vi "Add Crank Cam RTM Dependency.vi"(8 "error in (no error)":errorcluster, 9 "Menu hierarchy in":string[](array[string]), 11 "Node Ptr":u64 format="%.0x") -> (0 "error out":errorcluster, 1 "Menu hierarchy out":string[](array[string]), 3 "Action":T1)   [LabVIEW 2011, in "Engine Sim System Explorer.lvlib"]
uses:
  Engine Sim System Explorer.lvlib
  <vilib>/NI Veristand/Custom Device API/Custom Device RTM Dependency.ctl
  TypeDefs/NTeethComp.ctl
  TypeDefs/FullyCustomComp.ctl
  Shared/FullyCustomCommMode.ctl
  TypeDefs/FullyCustomProfilesComp.ctl
  Shared/Engine Simulation Global.vi
  <vilib>/NI Veristand/Custom Device API/Get Item Property (Variant).vi
  <vilib>/NI Veristand/Custom Device API/Custom Device API.lvlib
  Engine Simulation Shared.lvlib
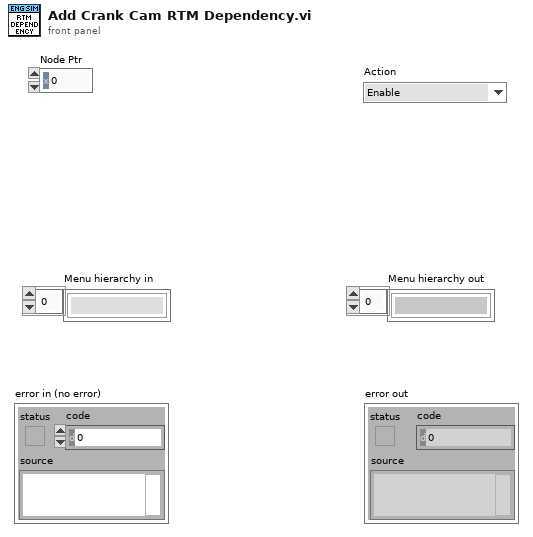
[diagram p1: front panel]
types:
  T1 = typedef "Custom Device API.lvlib/Custom Device RTM Dependency.ctl" = enum16{"Enable", "Disable", "Hide"}
  T2 = typedef "Engine Sim System Explorer.lvlib/FullyCustomComp.ctl" = cluster{"Name":string, "Comm Mode":T3, "Profiles":T4[]}
  T3 = typedef "Engine Simulation Shared.lvlib/FullyCustomCommMode.ctl" = enum16{"DMA FIFO", "FP Data Transfer"}
  T4 = typedef "Engine Sim System Explorer.lvlib/FullyCustomProfilesComp.ctl" = cluster{"Name":string, "Offset?":bool}
  T5 = typedef "Engine Sim System Explorer.lvlib/NTeethComp.ctl" = cluster{"Name":string, "TDC Offset":bool}
  T6 = typedef "Custom Device API.lvlib/Custom Device Item Ref.ctl" = u64
  T7 = typedef "Engine Sim System Explorer.lvlib/DataReplayLoopComp.ctl" = cluster{"Name":string, "DataReplays":T8[]}
  T8 = typedef "Engine Sim System Explorer.lvlib/DataReplayComp.ctl" = cluster{"Name":string, "Number":i32, "Optionals":bool[]}
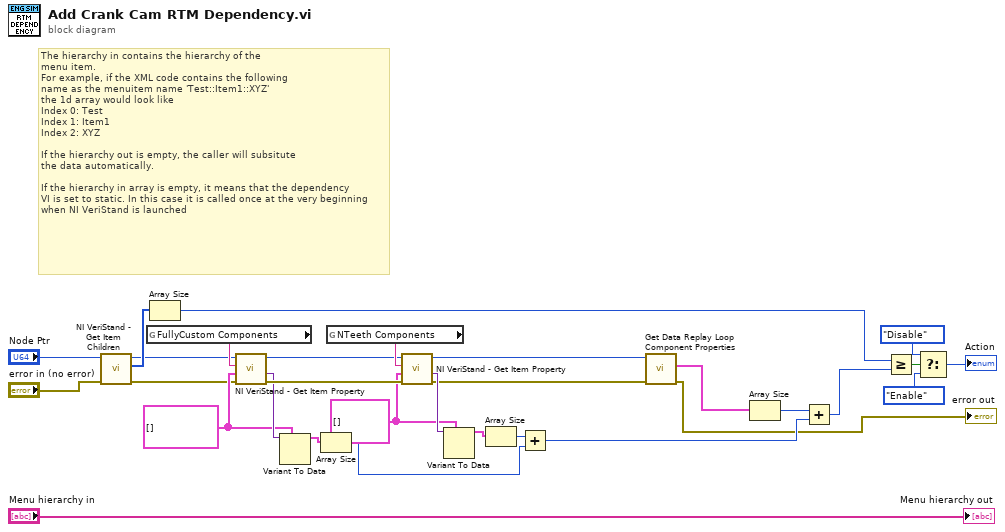
[diagram p0: block diagram]
diagram:
  w21 = T2[] []
  w19 = T5[] []
  # "The hierarchy in contains the hierarchy of the\nmenu item.\nFor example, if the XML code contains the following\nname as the menuitem name 'Test::Item1::XYZ'\nthe 1d array would look like\nIndex 0: Test\nIndex 1: Item1\nIndex 2: XYZ\n\nIf the hierarchy out is empty, the caller will subsitute\nthe data automatically.\n\nIf the hierarchy in array is empty, it means that the dependency\nVI is set to static. In this case it is called once at the very beginning\nwhen NI VeriStand is launched"
  n1 = call <vilib>:"NI VeriStand - Get Item Children.vi"("error in (no error)"="error in (no error)", "Item Ref in"="Node Ptr") -> ("error out"=w13:errorcluster, "Child Refs"=w28:T6[], "Item Ref out"=w14:T6)  [unwired: 6 in, 1 out]
  n2 = global read "Engine Simulation Global.vi" "FullyCustom Components"() -> (w26:string)
  n3 = Array Size(array=w28) -> (size(s)=w12:i32)
  n4 = call-poly <vilib>:"NI VeriStand - Get Item Property.vi"("error in (no error)"=w13, "Default Value"=w21, "Property Name"=w26, "Item Ref in"=w14) -> ("error out"=w23:errorcluster, "Value"=w22:variant, "Item Ref out"=w24:T6)  [unwired: 4 in, 1 out]
  n5 = Variant To Data(type=w21, Variant=w22) -> (data=w18:T2[])  [unwired: 1 in, 1 out]
  n6 = Array Size(array=w18) -> (size(s)=w15:i32)
  n7 = global read "Engine Simulation Global.vi" "NTeeth Components"() -> (w25:string)
  n8 = call-poly <vilib>:"NI VeriStand - Get Item Property.vi"("error in (no error)"=w23, "Default Value"=w19, "Property Name"=w25, "Item Ref in"=w24) -> ("error out"=w6:errorcluster, "Value"=w20:variant, "Item Ref out"=w7:T6)  [unwired: 4 in, 1 out]
  n9 = Variant To Data(type=w19, Variant=w20) -> (data=w17:T5[])  [unwired: 1 in, 1 out]
  n10 = Array Size(array=w17) -> (size(s)=w16:i32)
  n11 = Add(x=w16, y=w15) -> (x+y=w4:i32)
  n12 = call "Get Data Replay Loop Component Properties.vi"("error in (no error)"=w6, "Item Ref in"=w7) -> ("error out"=→"error out":errorcluster, "DataReplayLoops"=w1:T7[])  [unwired: 7 in, 1 out]
  n13 = Array Size(array=w1) -> (size(s)=w5:i32)
  n14 = Add(x=w5, y=w4) -> (x+y=w3:i32)
  n15 = Greater Or Equal?(x=w12, y=w3) -> (x >= y?=w11:bool)
  n16 = Select(t=Custom_Device_RTM_Dependency."Disable" ("Action"), s=w11, f=Custom_Device_RTM_Dependency."Enable" ("Action")) -> (s? t:f=→"Action":T1)
  "Menu hierarchy out" <- "Menu hierarchy in"
